vi "Write Ocean optics configuration.vi"(8 "error in (no error)":errorcluster, 10 "Rubi spectra configuration":T1={"Integration time"=0.5, "Fit parameters"={"Peaks"=[{"Amplitude"=4000.0, "Center"=694.3, "Width"=0.4}, {"Amplitude"=2000.0, "Center"=692.8, "Width"=0.4}], "Function"=enum."Gauss", "Window width"=0.0}, "Fit"=FALSE, "Auto-update params"=FALSE, "Save spectra"=FALSE} {"Fit parameters"."Window width" format="%#_6gnm"; "Fit parameters"."Peaks"."Width" format="%#_gnm"; "Fit parameters"."Peaks"."Center" format="%#_gnm"; "Integration time" format="%#_6ps"}, 11 "Ocean Optics Driver in":refnum<class "Ocean Optics Driver.lvclass">) -> (0 "error out":errorcluster, 3 "Ocean Optics Driver out":refnum<class "Ocean Optics Driver.lvclass">)   [LabVIEW 2016, in "Ocean Optics Driver.lvclass"]
uses:
  Ocean Optics Driver.lvclass
  C:/github/NHMFL_Core/Libraries/Instruments/Instrument Driver/Instrument Driver.lvclass
  Ocean optics configuration.ctl
  Utilities/Fit/Multi-peak Parameters.ctl
  Utilities/Fit/Peak Parameters.ctl
  Instrument Driver/Write User configuration.vi
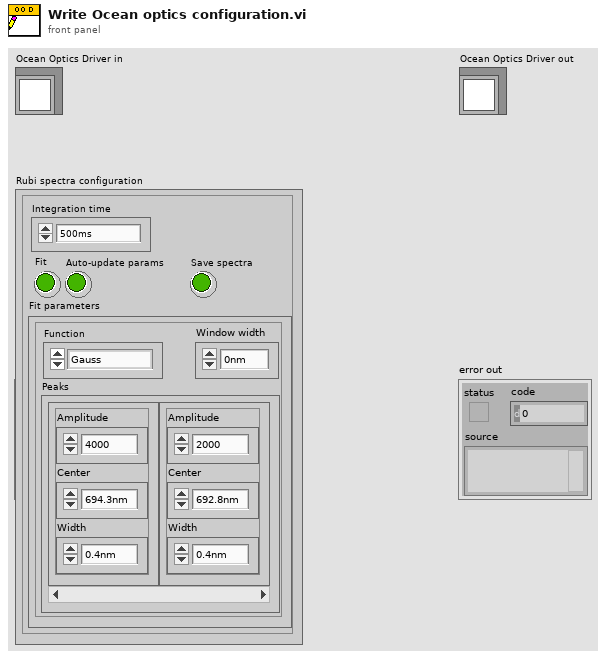
[diagram p1: front panel]
types:
  T1 = typedef "Ocean optics configuration.ctl" = cluster{"Integration time":dbl, "Fit parameters":T2, "Fit":bool, "Auto-update params":bool, "Save spectra":bool}
  T2 = typedef "Multi-peak Parameters.ctl" = cluster{"Peaks":T3[], "Function":enum16{"Gauss", "Lorentz"}, "Window width":dbl}
  T3 = typedef "Peak Parameters.ctl" = cluster{"Amplitude":dbl, "Center":dbl, "Width":dbl}
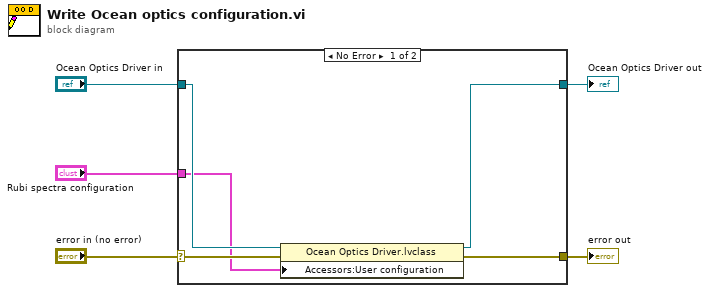
[diagram p0: block diagram]
diagram:
  n1 = case shown="No Error" "error in (no error)" {
    selector: "error in (no error)" -> [w10 w11]
    tunnel: [w9 w11] -> w4
    tunnel: [w7 w12] -> w2
    tunnel: "Ocean Optics Driver in" -> [w8 w12]
    tunnel: "Rubi spectra configuration" -> [w6 _]
    frame No Error {
      n2 = property class="Ocean Optics Driver.lvclass"(reference=w8, error in=w10, "Accessors:User configuration"=w6) -> (reference out=w7:refnum<class "Ocean Optics Driver.lvclass">, error out=w9:errorcluster)
    }
    frame Error {
    }
  }
  "error out" <- w4
  "Ocean Optics Driver out" <- w2
